vi "$TXSQ.vi"(10 "电文内容":string, 11 "用户地址":string) -> (2 "字符串":string, 3 "输出数组":u8[](array[numeric]) format="%02xH")   [LabVIEW 2016, in "环境动力监测库.lvlib" / "NMEA.lvlib"]
uses:
  NMEA.lvlib
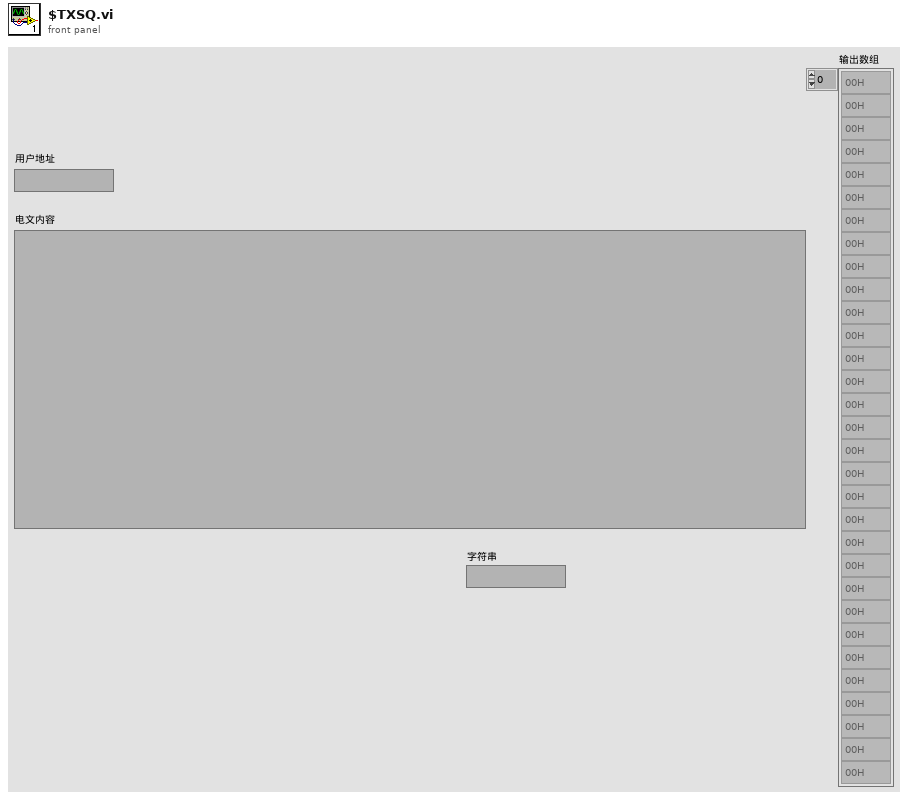
[diagram p1: front panel]
types:
  T1 = cluster{"指令/内容":string, "用户地址":string, "信息内容":u8[]}
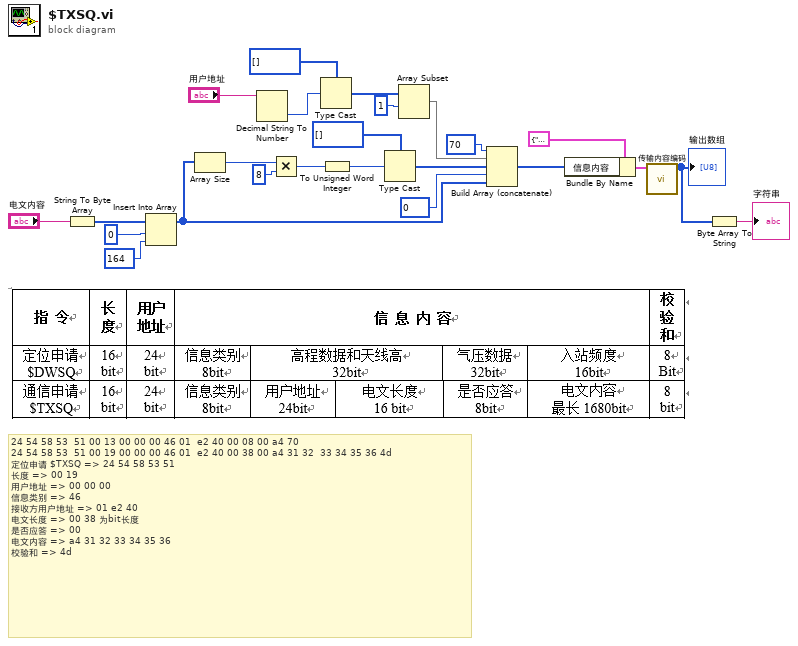
[diagram p0: block diagram]
diagram:
  # "24 54 58 53  51 00 13 00 00 00 46 01  e2 40 00 08 00 a4 70\n24 54 58 53  51 00 19 00 00 00 46 01  e2 40 00 38 00 a4 31 32  33 34 35 36 4d\n定位申请 $TXSQ => 24 54 58 53 51\n长度 => 00 19\n用户地址 => 00 00 00\n信息类别 => 46\n接收方用户地址 => 01 e2 40\n电文长度 => 00 38 为bit长度\n是否应答 => 00\n电文内容 => a4 31 32 33 34 35 36\n校验和 => 4d"
  n1 = String To Byte Array(string="电文内容") -> (unsigned byte array=w7:u8[])
  n2 = Insert Into Array(array=w7, index=0 ("索引"), new element=u8 164) -> (w4:u8[])
  n3 = Array Size(array=w4) -> (size(s)=w3:i32)
  n4 = Decimal String To Number(string="用户地址") -> (number=w20:i32)  [unwired: 2 in, 1 out]
  n5 = Multiply(x=w3, y=8) -> (x*y=w13:i32)
  n6 = Type Cast(type=u8[] [], x=w20) -> (*(type *) &x=w18:u8[])
  n7 = To Unsigned Word Integer(number=w13) -> (unsigned 16bit integer=w12:u16)
  n8 = Type Cast(type=u8[] [], x=w12) -> (*(type *) &x=w10:u8[])
  n9 = Array Subset(array=w18, index=1 ("索引")) -> (w15:u8[])  [unwired: 1 in]
  n10 = Build Array (concatenate)(u8 70, w15, w10, u8 0, w4) -> (w21:u8[])
  n11 = Bundle By Name(cluster=T1 {"指令/内容"="$TXSQ", "用户地址"="", "信息内容"=[]} ("输入"), "信息内容"=w21) -> (w23:T1)
  n12 = call "传输内容编码.vi"("输入"=w23) -> ("输出数组"=w2:u8[])  [unwired: 10 in]
  "输出数组" <- w2
  n13 = Byte Array To String(unsigned byte array=w2) -> (string=→"字符串":string)
